vi "BinFIFO.vi"(2 "HydraHarp":bool, 3 "binning (s)":dbl=0.01 format="%.2f", 4 "rawdata":T1) -> (0 "Counts":u32[](array[numeric]), 1 "MCS":u32[][](array[numeric]))   [LabVIEW 2009]
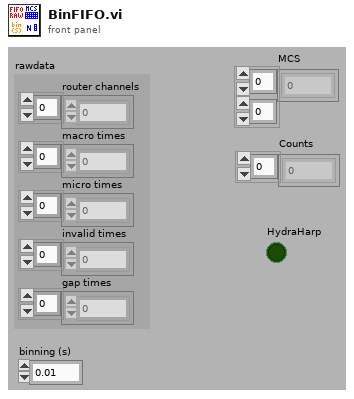
[diagram p1: front panel]
types:
  T1 = cluster{"router channels":u8[], "macro times":u32[], "micro times":u16[], "invalid times":u32[], "gap times":u32[]}
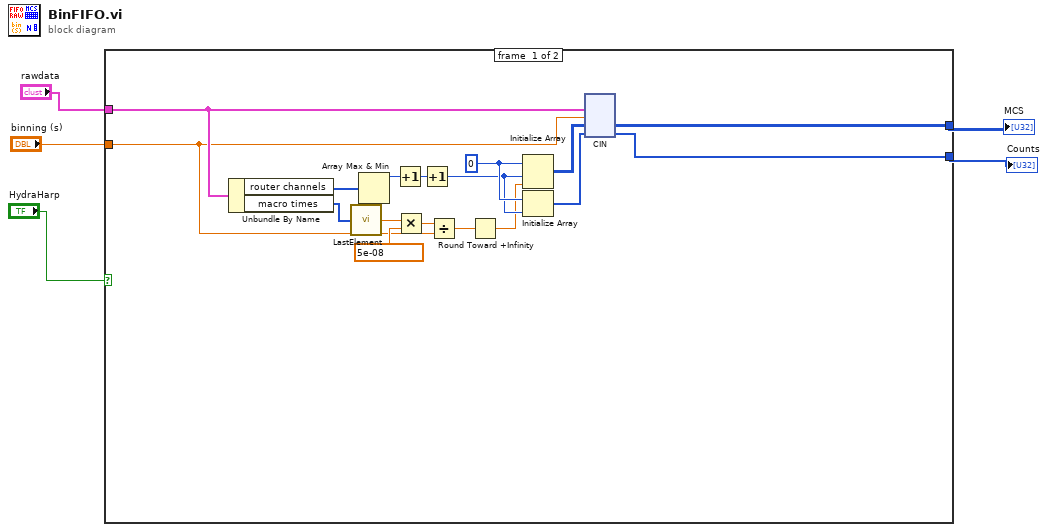
[diagram p0: block diagram]
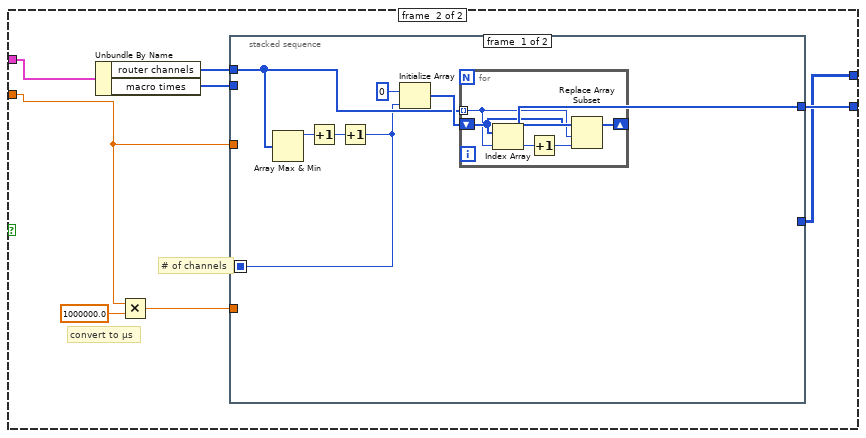
[diagram p2: hidden frame]
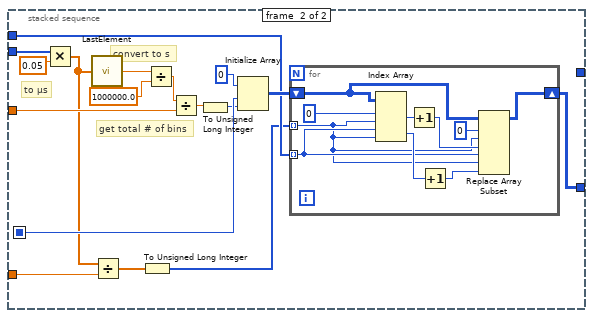
[diagram p3: hidden frame]
diagram:
  n1 = case shown="True" "HydraHarp" {
    tunnel: "rawdata" -> [w9 w30]
    tunnel: "binning (s)" -> [w8 w23]
    tunnel: [w7 w26] -> w3
    tunnel: [w6 w28] -> w2
    frame #0 {
      w18 = u32 0 ("element")
      n2 = Unbundle By Name(w9) -> ("router channels"=w11:u8[], "macro times"=w12:u32[])
      n3 = call "LastElement.vi"("array"=w12) -> ("Numeric"=w20:dbl)
      n4 = Array Max & Min(array=w11) -> (max value=w22:u8)  [unwired: 3 out]
      n5 = Increment(x=w22) -> (x+1=w21:u8)
      n6 = Multiply(x=w20, y=5e-08) -> (x*y=w14:dbl)
      n7 = Increment(x=w21) -> (x+1=w17:u8)
      n8 = Divide(x=w14, y=w8) -> (x/y=w13:dbl)
      n9 = Round Toward +Infinity(x=w13) -> (ceil(x): smallest int >= x=w10:dbl)
      n10 = Initialize Array(w18, w17, w10) -> (w19:u32[][])
      n11 = Initialize Array(w18, w17) -> (w16:u32[])
      n12 = cin(w9, w8, w19, w16) -> (w7:u32[][], w6:u32[])  [unwired: 2 in]
    }
    frame #1 {
      # "# of channels"
      # "convert to µs"
      n13 = Unbundle By Name(w30) -> ("router channels"=w29:u8[], "macro times"=w27:u32[])
      n14 = Multiply(x=w23, y=1000000.0) -> (x*y=w24:dbl)
      n15 = stacked-sequence {
        seq-local: [w31 _] -> [_ w55]
        tunnel: w29 -> [w34 w48]
        tunnel: [w35 _] -> w28
        tunnel: w27 -> [_ w43]
        tunnel: w24 -> [_ w47]
        tunnel: [_ w51] -> w26
        tunnel: w23 -> [_ w50]
        frame #0 {
          n16 = Array Max & Min(array=w34) -> (max value=w33:u8)  [unwired: 3 out]
          n17 = Increment(x=w33) -> (x+1=w32:u8)
          n18 = Increment(x=w32) -> (x+1=w31:u8)
          n19 = Initialize Array(u32 0 ("Element"), w31) -> (w36:u32[])
          n20 = for {
            tunnel: w34 -> [w39] mode=indexing
            shift-right: [w38] -> w35
            shift-left: w36 -> [w42]
            n21 = Index Array(array=w42, index=w39) -> (element=w41:u32)
            n22 = Increment(x=w41) -> (x+1=w40:u32)
            n23 = Replace Array Subset(array=w42, new element=w40, index=w39) -> (w38:u32[])
          }
        }
        frame #1 {
          # "to µs"
          # "get total # of bins"
          # "convert to s"
          n24 = Multiply(x=w43, y=0.05) -> (x*y=w46:dbl[])
          n25 = call "LastElement.vi"("array"=w46) -> ("Numeric"=w59:dbl)
          n26 = Divide(x=w46, y=w47) -> (x/y=w45:dbl[])
          n27 = To Unsigned Long Integer(number=w45) -> (unsigned 32bit integer=w44:u32[])
          n28 = Divide(x=w59, y=1000000.0) -> (x/y=w57:dbl)
          n29 = Divide(x=w57, y=w50) -> (x/y=w54:dbl)
          n30 = To Unsigned Long Integer(number=w54) -> (unsigned 32bit integer=w53:u32)
          n31 = Initialize Array(u32 0 ("Element"), w55, w53) -> (w52:u32[][])
          n32 = for {
            shift-right: [w62] -> w51
            shift-left: w52 -> [w65]
            tunnel: w48 -> [w61] mode=indexing
            tunnel: w44 -> [w60] mode=indexing
            n33 = Index Array(array=w65, index (row) #1=0 ("Index (Zeile)"), index (col) #1=w60, index (row) #2=w61, index (col) #2=w60) -> (element #1=w67:u32, element #2=w64:u32)
            n34 = Increment(x=w67) -> (x+1=w66:u32)
            n35 = Increment(x=w64) -> (x+1=w63:u32)
            n36 = Replace Array Subset(array=w65, new element #1=w66, index (row) #1=0 ("Deaktivierter Index (Zeile)"), index (col) #1=w60, new element #2=w63, index (row) #2=w61, index (col) #2=w60) -> (w62:u32[][])
          }
        }
      }
    }
  }
  "MCS" <- w3
  "Counts" <- w2
